vi "updateWaypoints.vi"(8 "error in (no error)":errorcluster, 11 "Drive in":refnum<class "Drive.lvclass">) -> (0 "error out":errorcluster, 3 "Drive out":refnum<class "Drive.lvclass">)   [LabVIEW 2011, in "Drive.lvclass"]
uses:
  Drive.lvclass
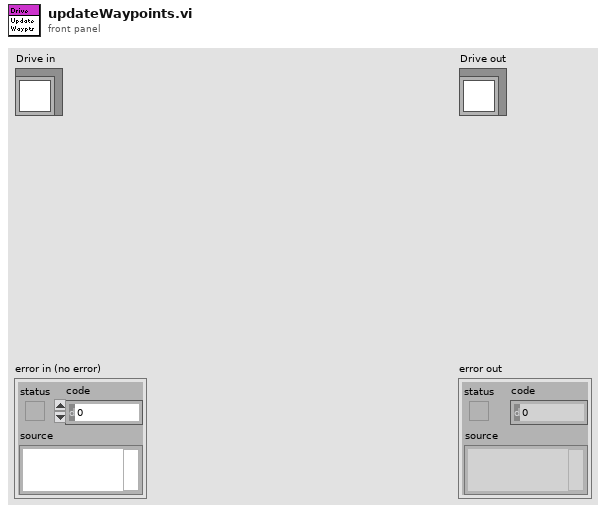
[diagram p1: front panel]
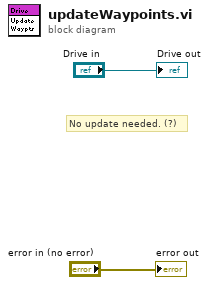
[diagram p0: block diagram]
diagram:
  # "No update needed. (?)"
  "error out" <- "error in (no error)"
  "Drive out" <- "Drive in"
